vi "sons.vi"(11 "Index Son":i16=1) -> ()   [LabVIEW 2019]
panel:
  in  "Son 4":path=path "C:/BonOMM_git/Config/Sons/4-Ouverture-windows.wav"
  in  "Son 3":path=path "C:/BonOMM_git/Config/Sons/3-fermeture-windows.wav"
  in  "Son 2":path=path "C:/BonOMM_git/Config/Sons/2-coups de vent.wav"
  in  "Son":path=path "C:/BonOMM_git/Config/Sons/1-alarme.wav"
  # "1 Son d'alarme"
  # "2 Son de coup de vent"
  # "3 Son Ouverture"
  # "4 Son Fermeture"
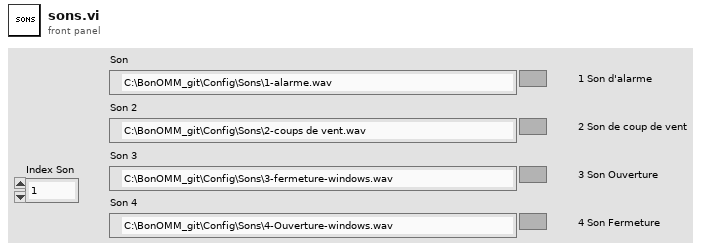
[diagram p1: front panel]
types:
  T1 = typedef "Sound Output Task ID.ctl" = u32
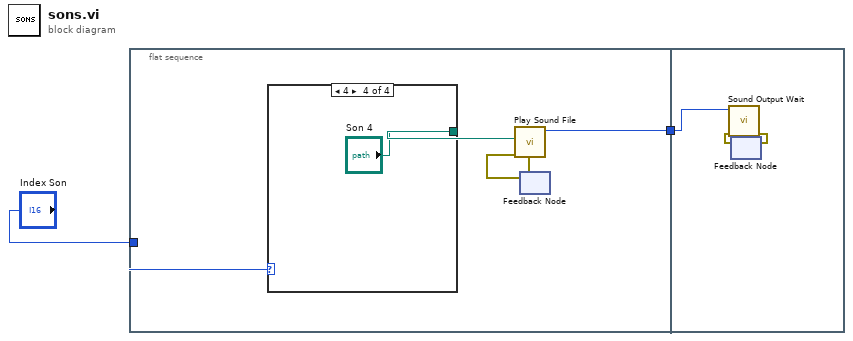
[diagram p0: block diagram]
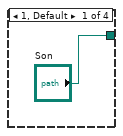
[diagram p2: hidden frame]
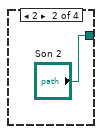
[diagram p3: hidden frame]
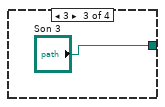
[diagram p4: hidden frame]
diagram:
  n1 = flat-sequence {
    tunnel: "Index Son" -> [w7]
    tunnel: [w3] -> w1
    tunnel: w1 -> [w14]
    frame #0 {
      n2 = case shown="4" w7 {
        tunnel: ["Son" "Son 2" "Son 3" "Son 4"] -> w6
        frame 1, Default {
        }
        frame 2 {
        }
        frame 3 {
        }
        frame 4 {
        }
      }
      n3 = feedback #1() -> (w4:errorcluster)  [unwired: 1 in]
      n4 = call <vilib>:"Play Sound File.vi"("error in (no error)"=w4, "path"=w6) -> ("error out"=w5:errorcluster, "task ID"=w3:T1)  [unwired: 8 in]
      n5 = feedback-in #1(w5) -> ()
    }
    frame #1 {
      n6 = feedback #2() -> (w12:errorcluster)  [unwired: 1 in]
      n7 = call <vilib>:"Sound Output Wait.vi"("error in (no error)"=w12, "task ID"=w14) -> ("error out"=w13:errorcluster)  [unwired: 8 in, 1 out]
      n8 = feedback-in #2(w13) -> ()
    }
  }
